vi "CheckMethodName.vi"(1 "Class Folder":path, 2 "Name":string, 3 "OriginalExtension":string, 4 "ClassName":string, 5 "error in (no error)":errorcluster) -> (15 "ValidName?":bool, 16 "Exists?":bool, 17 "Message":string, 19 "error out":errorcluster)   [LabVIEW 2020, in "G#IDE.lvlib" / "LibraryLib.lvlib"]
uses:
  LibraryLib.lvlib
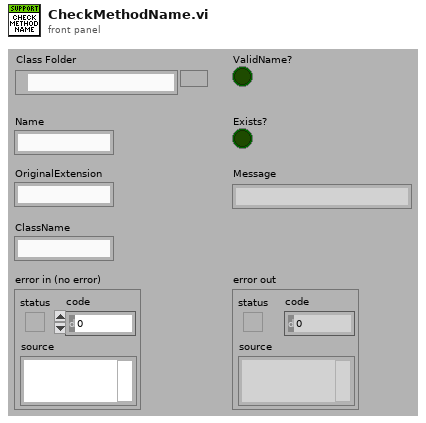
[diagram p1: front panel]
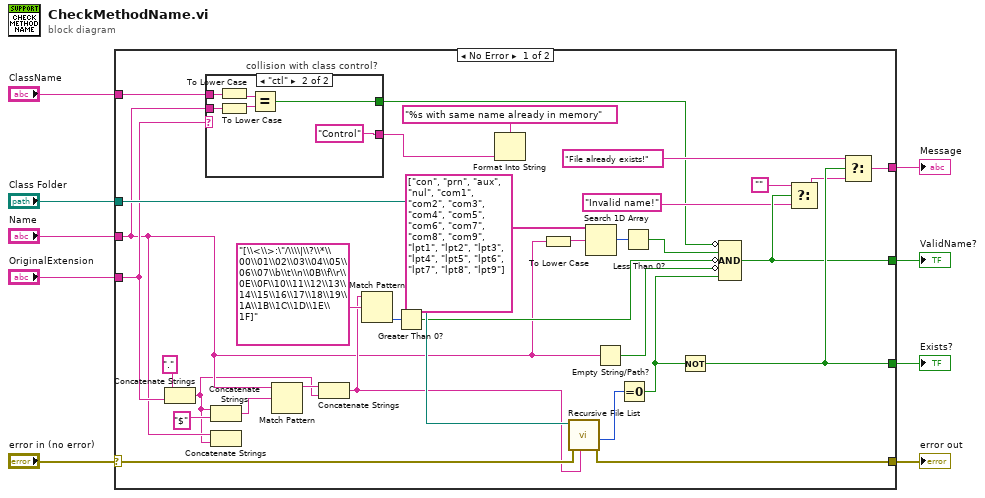
[diagram p0: block diagram]
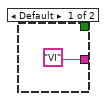
[diagram p2: hidden frame]
diagram:
  n1 = case shown="No Error" "error in (no error)" {
    selector: "error in (no error)" -> [w33 w49]
    tunnel: [w16 w49] -> w9
    tunnel: "Class Folder" -> [w34 _]
    tunnel: "Name" -> [w12 _]
    tunnel: [w22 _] -> w5
    tunnel: [w28 _] -> w4
    tunnel: "OriginalExtension" -> [w19 _]
    tunnel: [w10 _] -> w2
    tunnel: "ClassName" -> [w18 _]
    frame No Error {
      n2 = Concatenate Strings("." ("string"), w19) -> (w11:string)
      n3 = case "collision with class control?" shown="\"ctl\"" w19 {
        tunnel: w18 -> [_ w48]
        tunnel: w12 -> [_ w47]
        tunnel: [_ w44] -> w17
        tunnel: ["VI" "Control"] -> w14
        frame Default {
        }
        frame "ctl" {
          n4 = To Lower Case(string=w48) -> (all lower case string=w46:string)
          n5 = To Lower Case(string=w47) -> (all lower case string=w45:string)
          n6 = Equal?(x=w46, y=w45) -> (x = y?=w44:bool)
        }
      }
      n7 = Concatenate Strings(w11, "$" ("regular expression")) -> (w29:string)
      n8 = Concatenate Strings(w12, w11) -> ()  [unwired: 1 out]
      n9 = Match Pattern(string=w12, regular expression=w29) -> (before substring=w41:string)  [unwired: 4 out]
      n10 = Concatenate Strings(w41, w11) -> (w13:string)
      n11 = Match Pattern(string=w13, regular expression="[\\<\\>:\"/\\\\|\\?\\*\\00\\01\\02\\03\\04\\05\\06\\07\\b\\t\\n\\0B\\f\\r\\0E\\0F\\10\\11\\12\\13\\14\\15\\16\\17\\18\\19\\1A\\1B\\1C\\1D\\1E\\1F]") -> (offset past match=w25:i32)  [unwired: 1 in, 3 out]
      n12 = Greater Than 0?(x=w25) -> (x > 0?=w24:bool)
      n13 = Format Into String(format string="%s with same name already in memory", w14) -> ()  [unwired: 2 in, 2 out]
      n14 = To Lower Case(string=w12) -> (all lower case string=w39:string)
      n15 = call <vilib>:"Recursive File List.vi"("pattern"=w13, "error in (no error)"=w33, "Folder Path"=w34) -> ("error out"=w16:errorcluster, "Number of Files"=w37:i32)  [unwired: 4 in, 3 out]
      n16 = Search 1D Array(1D array=string[] ["con", "prn", "aux", "nul", "com1", "com2", "com3", "com4", "com5", "com6", "com7", "com8", "com9", "lpt1", "lpt2", "lpt3", "lpt4", "lpt5", "lpt6", "lpt7", "lpt8", "lpt9"], element=w39) -> (index of element=w38:i32)  [unwired: 1 in]
      n17 = Empty String/Path?(string/path=w12) -> (empty?=w35:bool)
      n18 = Equal To 0?(x=w37) -> (x = 0?=w32:bool)
      n19 = Less Than 0?(x=w38) -> (x < 0?=w36:bool)
      n20 = Not(x=w32) -> (.not. x?=w28:bool)
      n21 = Compound Arithmetic op=AND(invert w17, w36, invert w24, invert w35, w32) -> (w22:bool)
      n22 = Select(t="", s=w22, f="Invalid name!") -> (s? t:f=w23:string)
      n23 = Select(t="File already exists!", s=w28, f=w23) -> (s? t:f=w10:string)
    }
    frame Error {
    }
  }
  "error out" <- w9
  "ValidName?" <- w5
  "Exists?" <- w4
  "Message" <- w2
